vi "XIPIN_SMPTE_2022-1_2_Video_over_IP_Transmitter_2_0.vi"   [LabVIEW 2017]
doc: "The Xilinx LogiCORE IP SMPTE 2022-1/2 Video over IP Transmitter is a module for broadcast applications that requires bridging between SMPTE video connectivity standard (ASI) and 1 Gb/s networks. It is capable of mapping transport streams into Ethernet packets and adding systematically generated redundant data.\n------------------------------------\n<b>Need License</b> : Yes\n<b>Interface</b> : AXI4 AXI4-Stream"
uses:
  <vilib>/rvi/XilinxIP/XIPIN_XNode/niFpgaXIPIN.xnode
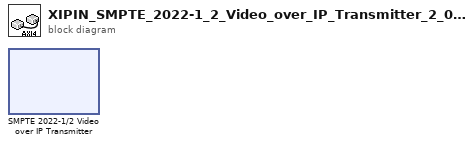
[diagram p0: block diagram]
diagram:
  n1 = xnode ("SMPTE 2022-1/2 Video over IP Transmitter")() -> ()
